vi "Magic Wand.vi"() -> ()   [LabVIEW 2014]
doc: "This example shows how to create an image mask by extracting a region surrounding a reference pixel, called the origin, and using a tolerance (+ or -) of intensity variations based on this reference pixel. Using this origin, the Magic Wand Tool searches for its neighbors with an intensity equal to or falling within the tolerance value of the point of reference."
uses:
  <vilib>/vision/NI_Vision_Development_Module.lvlib
panel:
  out "Magic Wand Result":T1(plugin-control)
  out "Image Source":T1(plugin-control)
  in  "Connectivity":bool
  in  "Tolerance":sgl=20.0
  in  "Stop":bool
  # "Overview: Demonstrates extract using an object in an image using the Magic Wand algorithm.\nRequirements: NI Vision Development Module\nInstructions: \n1. Run the VI. \n2. Click on the object you want to segment in the Image Source."
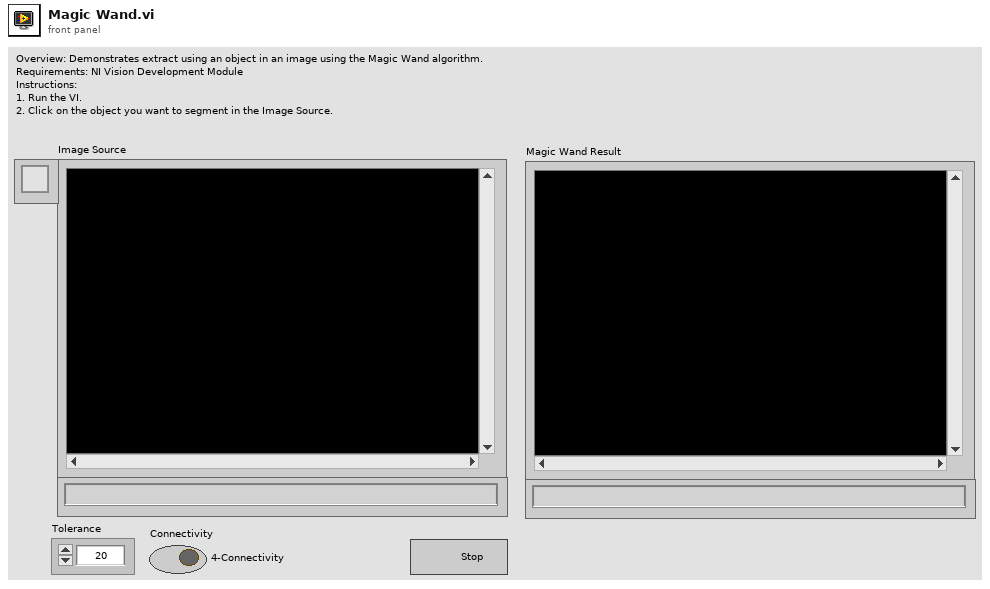
[diagram p1: front panel]
types:
  T1 = typedef "IMAQ Image.ctl" = refnum<image>
  T2 = typedef "Image Type" = u32
  T3 = typedef "ROI Descriptor" = cluster{"Global Rectangle":i32[], "Contours":cluster{"ID":enum32{"External", "Internal"}, "Type":u32, "Coordinates":i32[]}[]}
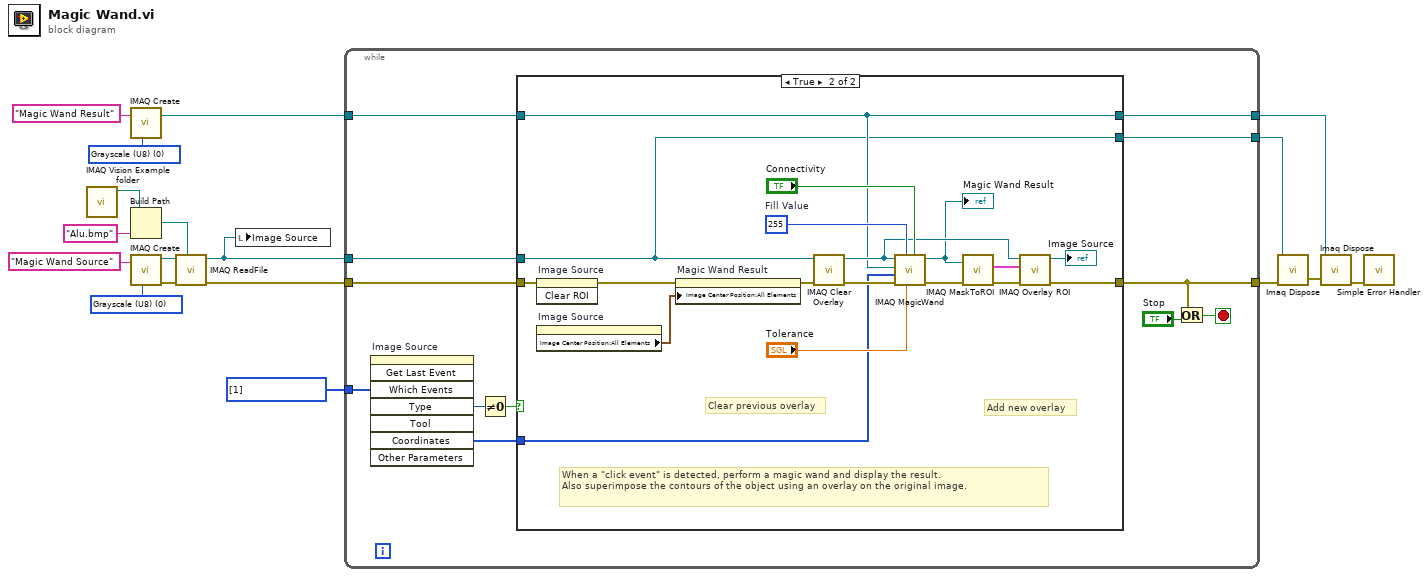
[diagram p0: block diagram]
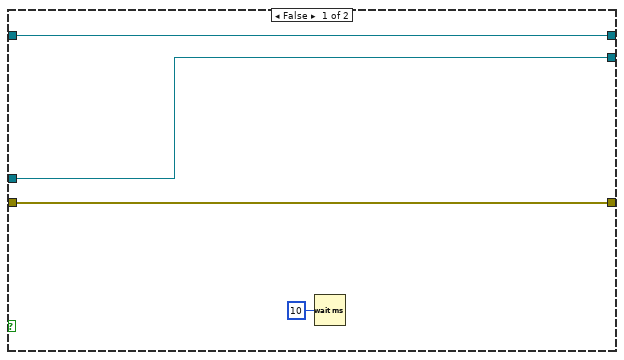
[diagram p2: hidden frame]
diagram:
  w3 = T2 0 items=["Grayscale (U8)", "Grayscale (I16)", "Grayscale (SGL)", "Complex (CSG)", "RGB (U32)", "HSL (U32)", "RGB (U64)", "Grayscale (U16)"] ("Image Type")
  w4 = T2 0 items=["Grayscale (U8)", "Grayscale (I16)", "Grayscale (SGL)", "Complex (CSG)", "RGB (U32)", "HSL (U32)", "RGB (U64)", "Grayscale (U16)"] ("Image Type")
  w11 = i32[] [1] items=["No  event", "Click event", "Draw event", "Move event", "Size event", "Scroll event", "Activate event", "Close event", "Double click event"] ("Events list (all)")
  n1 = call "IMAQ Vision Example folder.vi"() -> ("Example Image Path"=w16:path)  [unwired: 11 in]
  n2 = call "IMAQ Create"("Image Name"="Magic Wand Result", "Image Type"=w4) -> ("New Image"=w9:T1)  [unwired: 3 in, 1 out]
  n3 = Build Path(base path=w16, name or relative path="Alu.bmp") -> (appended path=w18:path)
  n4 = call "IMAQ Create"("Image Name"="Magic Wand Source", "Image Type"=w3) -> ("New Image"=w13:T1, "error out"=w12:errorcluster)  [unwired: 3 in]
  n5 = call "IMAQ ReadFile"("File Path"=w18, "error in (no error)"=w12, "Image"=w13) -> ("error out"=w10:errorcluster, "Image Out"=w8:T1)  [unwired: 4 in, 3 out]
  n6 = local write "Image Source"(w8) -> ()
  n7 = while {
    tunnel: w8 -> [w28]
    tunnel: w11 -> [w27]
    tunnel: w10 -> [w26]
    tunnel: w9 -> [w25]
    tunnel: [w21] -> w7
    tunnel: [w20] -> w2
    tunnel: [w19] -> w1
    stop <- w23 stop-if-true
    n8 = invoke on="Image Source" class="ImageControl" method="Get Last Event"("Which Events"=w27) -> ("Type"=w29:i32, "Coordinates"=w22:i32[])  [unwired: 7 in, 6 out]
    n9 = Not Equal To 0?(x=w29) -> (x != 0?=w30:bool)
    n10 = case shown="True" w30 {
      tunnel: w28 -> [w31 w36]
      tunnel: w26 -> [w33 w39]
      tunnel: w25 -> [w32 w37]
      tunnel: [w33 w44] -> w21
      tunnel: w22 -> [_ w35]
      tunnel: [w32 w37] -> w20
      tunnel: [w31 w36] -> w19
      frame False {
        n11 = Wait (ms)(milliseconds to wait=u32 10) -> ()  [unwired: 1 out]
      }
      frame True {
        w50 = u8 255  # Fill Value
        # "When a \"click event\" is detected, perform a magic wand and display the result.\nAlso superimpose the contours of the object using an overlay on the original image."
        # "Add new overlay"
        # "Clear previous overlay"
        n12 = invoke on="Image Source" class="ImageControl" method="Clear ROI"(error in=w39) -> (error out=w41:errorcluster)  [unwired: 2 in, 2 out]
        n13 = property on="Image Source" class="ImageControl"() -> ("Image Center Position:All Elements"=w42:cluster{"X":u32, "Y":u32})  [unwired: 2 in, 2 out]
        n14 = property on="Magic Wand Result" class="ImageControl"(error in=w41, "Image Center Position:All Elements"=w42) -> (error out=w40:errorcluster)  [unwired: 1 in, 1 out]
        n15 = call "IMAQ Clear Overlay"("error in (no error)"=w40, "Image"=w36) -> ("error out"=w47:errorcluster, "Image Out"=w45:T1)  [unwired: 8 in]
        n16 = call "IMAQ MagicWand"("Connectivity 4/8 (8)"="Connectivity", "Tolerance"="Tolerance", "Fill Value"=w50, "error in (no error)"=w47, "Hot spot (x,y)"=w35, "Image Dst"=w37, "Image Src"=w45) -> ("error out"=w46:errorcluster, "Image Dst Out"=w38:T1)  [unwired: 3 in]
        "Magic Wand Result" <- w38
        n17 = call "IMAQ MaskToROI"("Image"=w38, "error in (no error)"=w46) -> ("ROI Descriptor"=w48:T3, "error out"=w49:errorcluster)  [unwired: 5 in, 1 out]
        n18 = call "IMAQ Overlay ROI"("error in (no error)"=w49, "ROI Descriptor"=w48, "Image"=w45) -> ("error out"=w44:errorcluster, "Image Out"=→"Image Source":T1)  [unwired: 7 in]
      }
    }
    n19 = Or(x=w21, y="Stop") -> (x .or. y?=w23:bool)
  }
  n20 = call "Imaq Dispose"("Image"=w1, "error in (no error)"=w7) -> ("error out"=w6:errorcluster)  [unwired: 4 in]
  n21 = call "Imaq Dispose"("Image"=w2, "error in (no error)"=w6) -> ("error out"=w5:errorcluster)  [unwired: 4 in]
  n22 = call <vilib>:"Simple Error Handler.vi"("error in (no error)"=w5) -> ()  [unwired: 4 in, 5 out]
